vi "error.vi"(8 "error in":errorcluster, 11 "REST Response":string) -> (0 "error out":errorcluster)   [LabVIEW 2020, in "Nominal Client.lvclass"]
uses:
  Nominal Client.lvclass
  859f8e04-e495-489b-b5b4-7ac163f56130.vi
  <vilib>/JDP Science/JSONtext/JSON text to Variant.vi
  <vilib>/JDP Science/JSONtext/LVClass Serializer/JSONtext LVClass Serializer.lvclass
  <vilib>/JDP Science/JSONtext/JSONtext.lvlib
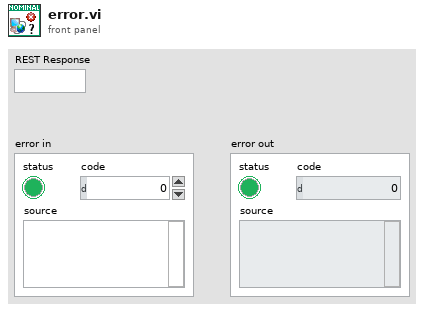
[diagram p1: front panel]
types:
  T1 = cluster{"errorCode":string, "errorName":string, "errorInstanceId":string}
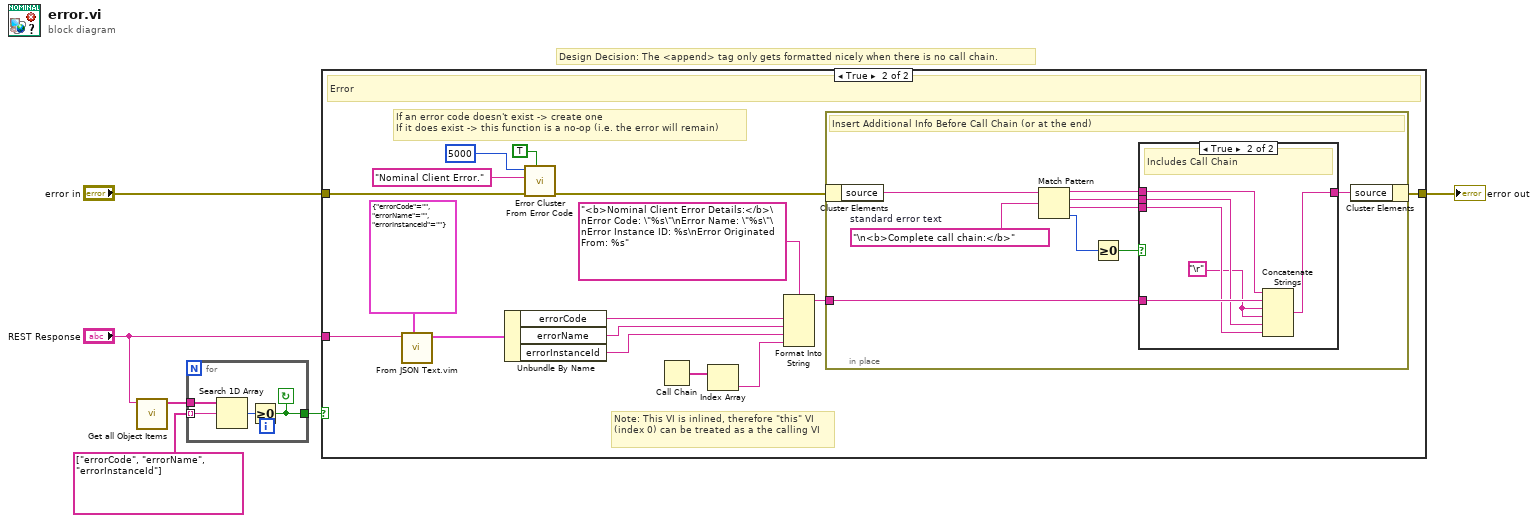
[diagram p0: block diagram]
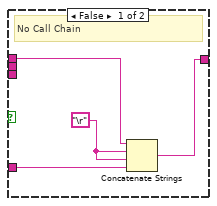
[diagram p3: hidden frame]
diagram:
  # "Design Decision: The <append> tag only gets formatted nicely when there is no call chain."
  n1 = call <vilib>:"Get all Object Items.vi"("JSON"="REST Response") -> ("Item Names"=w5:string[])  [unwired: 7 in, 3 out]
  n2 = for {
    tunnel: w5 -> [w10]
    tunnel: string[] ["errorCode", "errorName", "errorInstanceId"] ("Item Names") -> [w9] mode=indexing
    tunnel: [w7] -> w4
    stop <- w7 continue-if-true
    n3 = Search 1D Array(1D array=w10, element=w9) -> (index of element=w8:i32)  [unwired: 1 in]
    n4 = Greater Or Equal To 0?(x=w8) -> (x >= 0?=w7:bool)
  }
  n5 = case shown="True" w4 {
    tunnel: [w11 w24] -> w2
    tunnel: "REST Response" -> [_ w17]
    tunnel: "error in" -> [w11 w13]
    frame False {
      # "Not an error"
    }
    frame True {
      # "If an error code doesn't exist -> create one\nIf it does exist -> this function is a no-op (i.e. the error will remain)"
      # "Note: This VI is inlined, therefore \"this\" VI (index 0) can be treated as a the calling VI"
      # "Error"
      n6 = call "From JSON Text.vim"("Data Type and Default Value"=T1 {"errorCode"="", "errorName"="", "errorInstanceId"=""}, "JSON"=w17) -> ("Data out"=w22:T1)  [unwired: 8 in, 1 out]
      n7 = Unbundle By Name(w22) -> ("errorCode"=w20:string, "errorName"=w19:string, "errorInstanceId"=w18:string)
      n8 = call <vilib>:"Error Cluster From Error Code.vi"("show call chain? (False)"=TRUE, "error in (no error)"=w13, "error message (\"\")"="Nominal Client Error." ("error message (\"\")"), "error code (0)"=5000) -> ("error out"=w14:errorcluster)  [unwired: 5 in]
      n9 = Call Chain() -> (call chain=w27:string[])
      n10 = Index Array(array=w27) -> (element=w21:string)  [unwired: 1 in]
      n11 = Format Into String(format string="<b>Nominal Client Error Details:</b>\nError Code: \"%s\"\nError Name: \"%s\"\nError Instance ID: %s\nError Originated From: %s" ("search string"), w20, w19, w18, w21) -> (resulting string=w25:string)  [unwired: 2 in, 1 out]
      n12 = in-place {
        in-place-border: w25 -> [w35]
        w33 = "\n<b>Complete call chain:</b>"  # standard error text
        # "Insert Additional Info Before Call Chain (or at the end)"
        n13 = in-place-cluster #1(w14) -> ("source"=w34:string)
        n14 = Match Pattern(string=w34, regular expression=w33) -> (before substring=w30:string, match substring=w31:string, after substring=w32:string, offset past match=w29:i32)  [unwired: 1 in]
        n15 = Greater Or Equal To 0?(x=w29) -> (x >= 0?=w28:bool)
        n16 = case shown="True" w28 {
          tunnel: [w39 w46] -> w36
          tunnel: w35 -> [w37 w45]
          tunnel: w32 -> [_ w44]
          tunnel: w31 -> [_ w43]
          tunnel: w30 -> [w40 w42]
          frame False {
            w38 = "\r"
            # "No Call Chain"
            n17 = Concatenate Strings(w40, w38, w38, w37) -> (w39:string)
          }
          frame True {
            w41 = "\r"
            # "Includes Call Chain"
            n18 = Concatenate Strings(w42, w45, w41, w41, w43, w44) -> (w46:string)
          }
        }
        n19 = in-place-cluster #1("source"=w36) -> (w24:errorcluster)
      }
    }
  }
  "error out" <- w2
